vi "cal_objective_fun.vi"(3 "output control":T1, 4 "data":T2, 5 "X":dbl[](array[numeric])) -> (0 "error out":errorcluster, 1 "gradient":dbl[](array[numeric]), 2 "f(X)":dbl)   [LabVIEW 2014]
doc: "This template is the starting point for creating an objectivel function to be passed to the Unconstrained Optimization.vi."
uses:
  <vilib>/gmath/NumericalOptimization/objective function data.ctl
  <vilib>/gmath/NI_Gmath.lvlib
panel:
  out "X":dbl[][](graph)
  out "f(x)":dbl(graph)
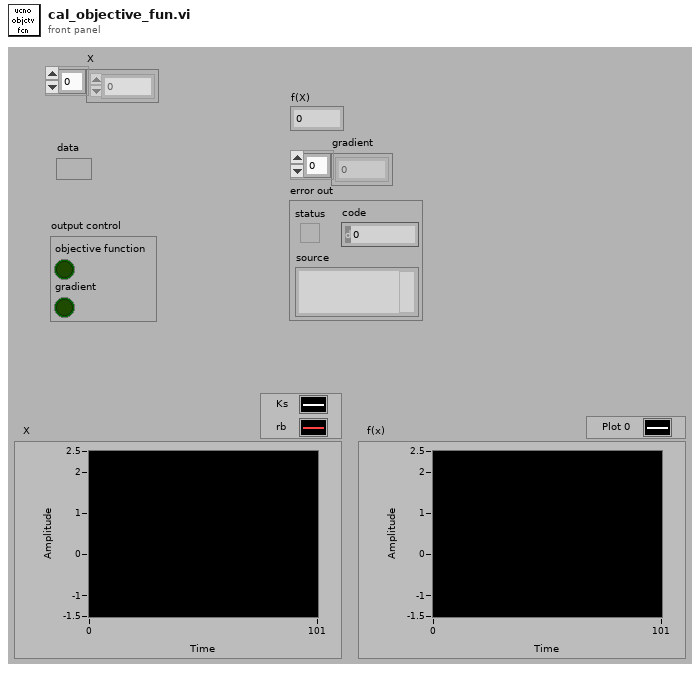
[diagram p1: front panel]
types:
  T1 = cluster{"objective function":bool, "gradient":bool}
  T2 = typedef "NI_Gmath.lvlib/objective function data.ctl" = variant
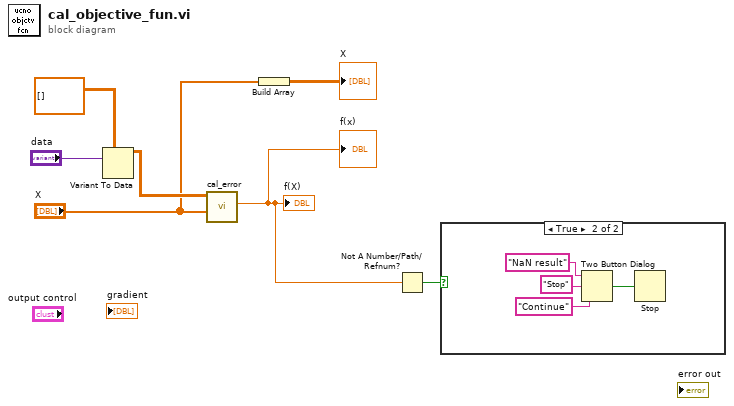
[diagram p0: block diagram]
diagram:
  n1 = Variant To Data(type=dbl[][] [] ("Cal data"), Variant="data") -> (data=w5:dbl[][])  [unwired: 1 in, 1 out]
  n2 = call "cal_error.vi"("X"="X", "Cal data"=w5) -> ("f(X)"=w3:dbl)  [unwired: 8 in, 1 out]
  "f(X)" <- w3
  "f(x)" <- w3
  n3 = Build Array("X") -> (→"X":dbl[][])
  n4 = Not A Number/Path/Refnum?(number/path/refnum=w3) -> (NaN/Path/Refnum?=w4:bool)
  n5 = case shown="True" w4 {
    frame False {
    }
    frame True {
      n6 = Two Button Dialog(message="NaN result", 1:"Continue" ("F button name (\"Cancel\")"), 2:"Stop" ("T button name (\"OK\")")) -> (T button?=w10:bool)
      n7 = Stop(stop? (T)=w10) -> ()
    }
  }
